vi "EF_DataProcThread.vi"(11 "EF_AllQRefs":T1) -> ()   [LabVIEW 2017]
uses:
  Types/EF_AllQRefs.ctl
  Types/EF_GUIThread_QRef.ctl
  Types/EF_GUIThread_QData.ctl
  Types/EF_GUIThread_QCmds.ctl
  Types/EF_DAQThread_QRef.ctl
  Types/EF_DAQThread_QData.ctl
  Types/EF_DAQThread_QCmds.ctl
  Types/EF_DataProcThread_QRef.ctl
  Types/EF_DataProcThread_QData.ctl
  Types/EF_DataProcThread_QCmds.ctl
  Types/EF_AnalysisThread_QRef.ctl
  Types/EF_AnalysisThread_QData.ctl
  Types/EF_AnalysisThread_QCmds.ctl
  Types/EF_DataProcThread_Data.ctl
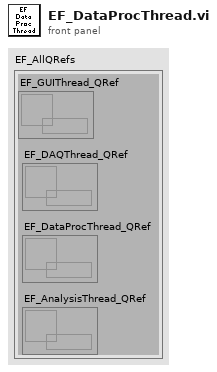
[diagram p1: front panel]
types:
  T1 = typedef "EF_AllQRefs.ctl" = cluster{"EF_GUIThread_QRef":T2, "EF_DAQThread_QRef":T3, "EF_DataProcThread_QRef":T4, "EF_AnalysisThread_QRef":T5}
  T2 = typedef "EF_GUIThread_QRef.ctl" = refnum<queue>
  T3 = typedef "EF_DAQThread_QRef.ctl" = refnum<queue>
  T4 = typedef "EF_DataProcThread_QRef.ctl" = refnum<queue>
  T5 = typedef "EF_AnalysisThread_QRef.ctl" = refnum<queue>
  T6 = typedef "EF_DataProcThread_Data.ctl" = cluster{"TimeTrace":u32[], "Histo":u32[], "Total bin":u64, "aboveThres":bool, "HistToZero":bool, "Bin":i32, "shift":i16, "Threshold":u32, "TotalBinHistStart":u64}
  T7 = typedef "EF_AnalysisThread_QData.ctl" = cluster{"Cmd":T8, "Histo":u32[], "DecayT0":dbl, "HistoRes":dbl, "TotalBinHistStart":u64, "TimeTraceRes":dbl, "Total bin":u64, "TickCount":u32, "LTThreshold":dbl, "TTLActivate":bool, "TTLDelay":dbl, "TTLWidth":dbl, "MinIntCounts":u32}
  T8 = typedef "EF_AnalysisThread_QCmds.ctl" = enum16{"Exit", "CalcAvgLT", "CalcDelay", "SetDecayT0", "SetHistoRes", "SetTimeTraceRes", "SetLTThreshold", "SetTTLActiv", "SetTTLDelay", "SetTTLWidth", "SetMinIntCounts"}
  T9 = typedef "EF_GUIThread_QCmds.ctl" = enum16{"_none_", "Res", "Histo", "TTrace", "Lifetime", "Rates", "Status", "ShortDelay", "_Error_"}
  T10 = typedef "EF_DataProcThread_QData.ctl" = cluster{"EF_DataProc_Cmds":T11, "nActual":i32, "Buffer":u32[], "TickCount":u32, "Param":i32}
  T11 = typedef "EF_DataProcThread_QCmds.ctl" = enum16{"Exit", "Proc", "Init", "SetShift", "SetThres"}
  T12 = typedef "EF_GUIThread_QData.ctl" = cluster{"Histo":u32[], "Rates":i32[], "Cmd":T9, "Res":dbl, "TimeTrace":u32[], "Bin":i32, "Status":string, "Total bin":u64, "AvgLTs":dbl[], "TotalBinsHistStart":u64[], "HistStartTimes":dbl[], "MinDelays":dbl[], "ShortDelay":bool, "Pending TTLs":i32, "error in (no error)":errorcluster, "DeltaT":dbl, "NumLTs":i32}
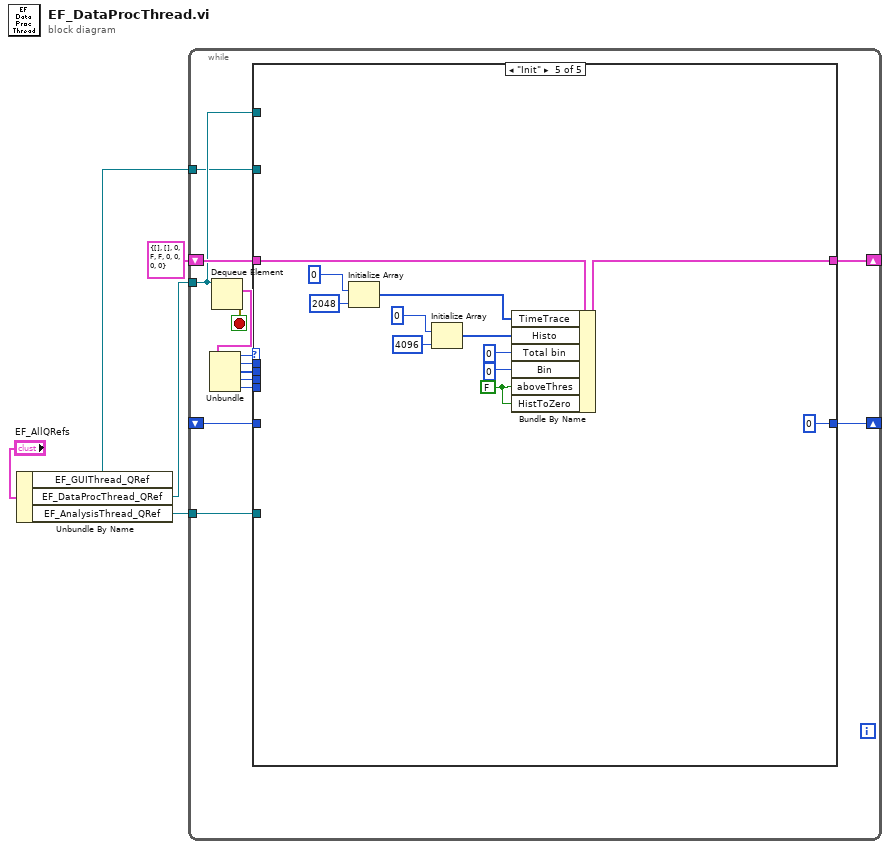
[diagram p0: block diagram]
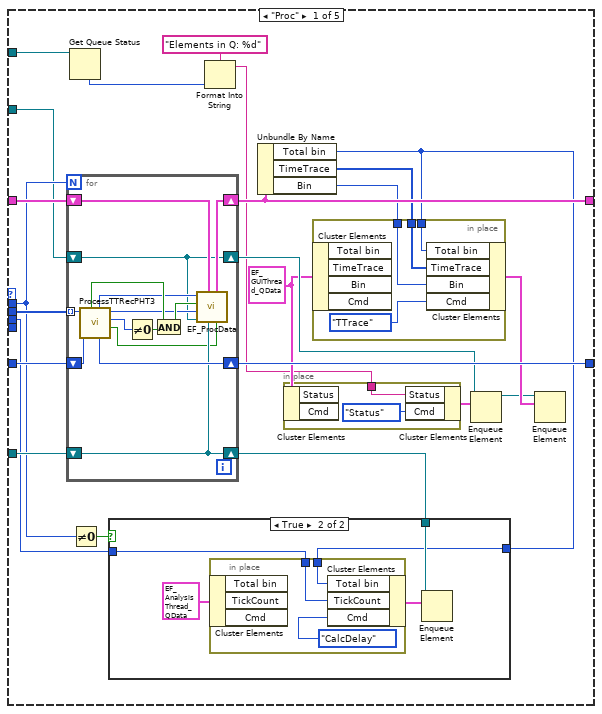
[diagram p2: hidden frame]
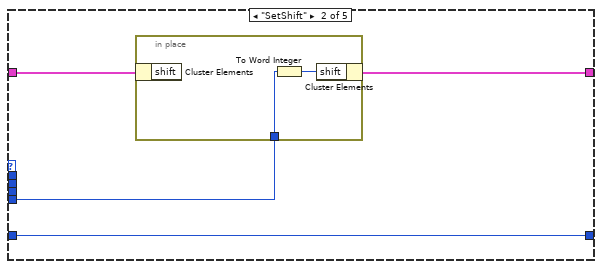
[diagram p4: hidden frame]
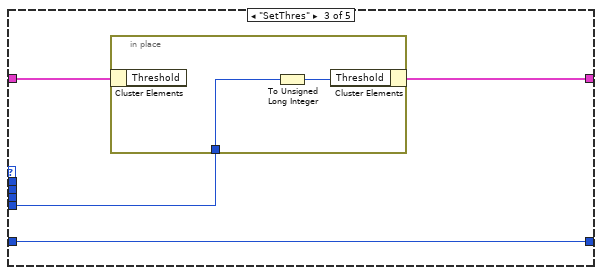
[diagram p5: hidden frame]
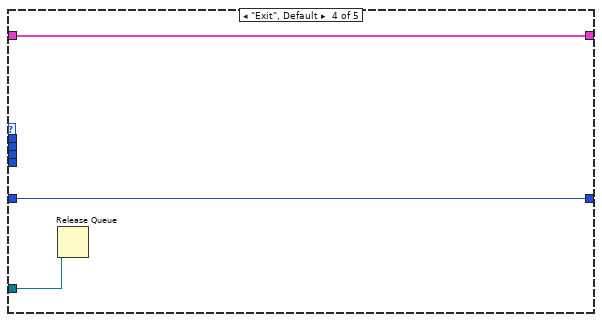
[diagram p6: hidden frame]
diagram:
  n1 = Unbundle By Name("EF_AllQRefs") -> ("EF_GUIThread_QRef"=w1:T2, "EF_DataProcThread_QRef"=w3:T4, "EF_AnalysisThread_QRef"=w2:T5)
  n2 = while {
    tunnel: w3 -> [w8]
    shift-right: [w15] -> _
    shift-left: _ -> [w14]
    shift-right: [w13] -> _
    shift-left: T6 {"TimeTrace"=[], "Histo"=[], "Total bin"=0, "aboveThres"=FALSE, "HistToZero"=FALSE, "Bin"=0, "shift"=0, "Threshold"=0, "TotalBinHistStart"=0} ("RTData_out") -> [w12]
    tunnel: w2 -> [w7]
    tunnel: w1 -> [w6]
    stop <- w11 stop-if-true
    n3 = Dequeue Element(queue=w8) -> (element=w19:T10, error out=w11:errorcluster)  [unwired: 2 in, 2 out]
    n4 = Unbundle(w19) -> ("EF_DataProc_Cmds"=w18:T11, "nActual"=w17:i32, "Buffer"=w16:u32[], "TickCount"=w10:u32, "Param"=w9:i32)
    n5 = case shown="\"Init\"" w18 {
      tunnel: w17 -> [w23 _ _ _ _]
      tunnel: w16 -> [w40 _ _ _ _]
      tunnel: [w42 w74 w80 w84 u64 0 ("ofl out")] -> w15
      tunnel: w14 -> [w41 w74 w80 w84 _]
      tunnel: [w39 w72 w77 w85 w87] -> w13
      tunnel: w12 -> [w26 w73 w79 w85 w86]
      tunnel: w10 -> [w24 _ _ _ _]
      tunnel: w9 -> [_ w71 w78 _ _]
      tunnel: w7 -> [w38 _ _ w83 _]
      tunnel: w8 -> [w34 _ _ _ _]
      tunnel: w6 -> [w20 _ _ _ _]
      frame "Proc" {
        w29 = T12 {"Histo"=[], "Rates"=[], "Cmd"=enum."_none_", "Res"=0.0, "TimeTrace"=[], "Bin"=0, "Status"="", "Total bin"=0, "AvgLTs"=[], "TotalBinsHistStart"=[], "HistStartTimes"=[], "MinDelays"=[], "ShortDelay"=FALSE, "Pending TTLs"=0, "error in (no error)"={"status"=FALSE, "code"=0, "source"=""}, "DeltaT"=0.0, "NumLTs"=0} ("element")
        n6 = for {
          N: w23 -> [_]
          tunnel: w40 -> [w64] mode=indexing
          shift-right: [w66] -> w42
          shift-left: w41 -> [w65]
          shift-right: [w63] -> w39
          shift-left: w26 -> [w60]
          shift-right: [w59] -> w31
          shift-left: w20 -> [w59]
          shift-right: [w58] -> w25
          shift-left: w38 -> [w58]
          n7 = call "ProcessTTRecPHT3.vi"("oflcorr_in"=w65, "rawbits"=w64) -> ("is_marker"=w57:bool, "channel"=w69:u32, "dtime"=w61:u32, "oflcorr_out"=w66:u64, "truetime"=w62:u64, "is_photon"=w68:bool)  [unwired: 3 in, 1 out]
          n8 = Not Equal To 0?(x=w69) -> (x != 0?=w70:bool)
          n9 = And(x=w68, y=w70) -> (x .and. y?=w67:bool)
          n10 = call "EF_ProcData.vi"("isMarker"=w57, "EF_AnalysisThread_QRef"=w58, "EFData in"=w60, "EF_GUIThread_QRef"=w59, "dtime"=w61, "photon&chan1"=w67, "truetime"=w62) -> ("EFData out"=w63:T6)  [unwired: 4 in]
        }
        n11 = Get Queue Status(queue=w34) -> (# elements in queue=w33:i32)  [unwired: 2 in, 7 out]
        n12 = Not Equal To 0?(x=w23) -> (x != 0?=w22:bool)
        n13 = Format Into String(format string="Elements in Q: %d", w33) -> (resulting string=w28:string)  [unwired: 2 in, 1 out]
        n14 = Unbundle By Name(w39) -> ("Total bin"=w21:u64, "TimeTrace"=w37:u32[], "Bin"=w36:i32)
        n15 = case shown="True" w22 {
          tunnel: w25 -> [_ w47]
          tunnel: w21 -> [_ w45]
          tunnel: w24 -> [_ w43]
          frame False {
          }
          frame True {
            n16 = in-place {
              in-place-border: w45 -> [w49]
              in-place-border: w43 -> [w48]
              n17 = in-place-cluster #1(T7 {"Cmd"=enum."CalcDelay", "Histo"=[], "DecayT0"=0.0, "HistoRes"=0.0, "TotalBinHistStart"=0, "TimeTraceRes"=0.0, "Total bin"=0, "TickCount"=0, "LTThreshold"=0.0, "TTLActivate"=FALSE, "TTLDelay"=0.0, "TTLWidth"=0.0, "MinIntCounts"=0} ("element")) -> ()  [unwired: 3 out]
              n18 = in-place-cluster #1("Total bin"=w49, "TickCount"=w48, "Cmd"=EF_AnalysisThread_QCmds."CalcDelay") -> (w44:T7)
            }
            n19 = Enqueue Element(queue=w47, element=w44) -> ()  [unwired: 2 in, 3 out]
          }
        }
        n20 = in-place {
          in-place-border: w28 -> [w51]
          n21 = in-place-cluster #2(w29) -> ()  [unwired: 2 out]
          n22 = in-place-cluster #2("Status"=w51, "Cmd"=EF_GUIThread_QCmds."Status") -> (w27:T12)
        }
        n23 = in-place {
          in-place-border: w37 -> [w56]
          in-place-border: w36 -> [w55]
          in-place-border: w21 -> [w53]
          n24 = in-place-cluster #3(w29) -> ()  [unwired: 4 out]
          n25 = in-place-cluster #3("Total bin"=w53, "TimeTrace"=w56, "Bin"=w55, "Cmd"=EF_GUIThread_QCmds."TTrace") -> (w35:T12)
        }
        n26 = Enqueue Element(queue=w31, element=w27) -> (queue out=w30:T2)  [unwired: 2 in, 2 out]
        n27 = Enqueue Element(queue=w30, element=w35) -> ()  [unwired: 2 in, 3 out]
      }
      frame "SetShift" {
        n28 = in-place {
          in-place-border: w71 -> [w76]
          n29 = in-place-cluster #4(w73) -> ()  [unwired: 1 out]
          n30 = To Word Integer(number=w76) -> (16bit integer=w75:i16)
          n31 = in-place-cluster #4("shift"=w75) -> (w72:T6)
        }
      }
      frame "SetThres" {
        n32 = in-place {
          in-place-border: w78 -> [w82]
          n33 = in-place-cluster #5(w79) -> ()  [unwired: 1 out]
          n34 = To Unsigned Long Integer(number=w82) -> (unsigned 32bit integer=w81:u32)
          n35 = in-place-cluster #5("Threshold"=w81) -> (w77:T6)
        }
      }
      frame "Exit", Default {
        n36 = Release Queue(queue=w83) -> ()  [unwired: 2 in, 3 out]
      }
      frame "Init" {
        w88 = FALSE ("above thres")
        n37 = Initialize Array(u32 0, 2048 ("dimension size")) -> (w94:u32[])
        n38 = Initialize Array(u32 0, 4096 ("dimension size")) -> (w91:u32[])
        n39 = Bundle By Name(cluster=w86, "TimeTrace"=w94, "Histo"=w91, "Total bin"=u64 0 ("Last total bin"), "Bin"=0 ("Last bin"), "aboveThres"=w88, "HistToZero"=w88) -> (w87:T6)
      }
    }
  }
